vi "register status change event.vi"(11 "generate status number":i32=100) -> (3 "status number":i32)   [LabVIEW 2017, in "testcase-Basic-Function.lvclass"]
uses:
  testcase-Basic-Function.lvclass
  f9bca660-bddd-4266-99d8-d96952150cc2.vi
  src/user.lib/_NEVSTOP/Communicable State Machine(CSM)/Communicable State Machine.lvlib
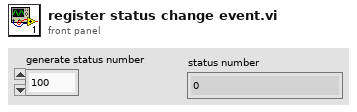
[diagram p1: front panel]
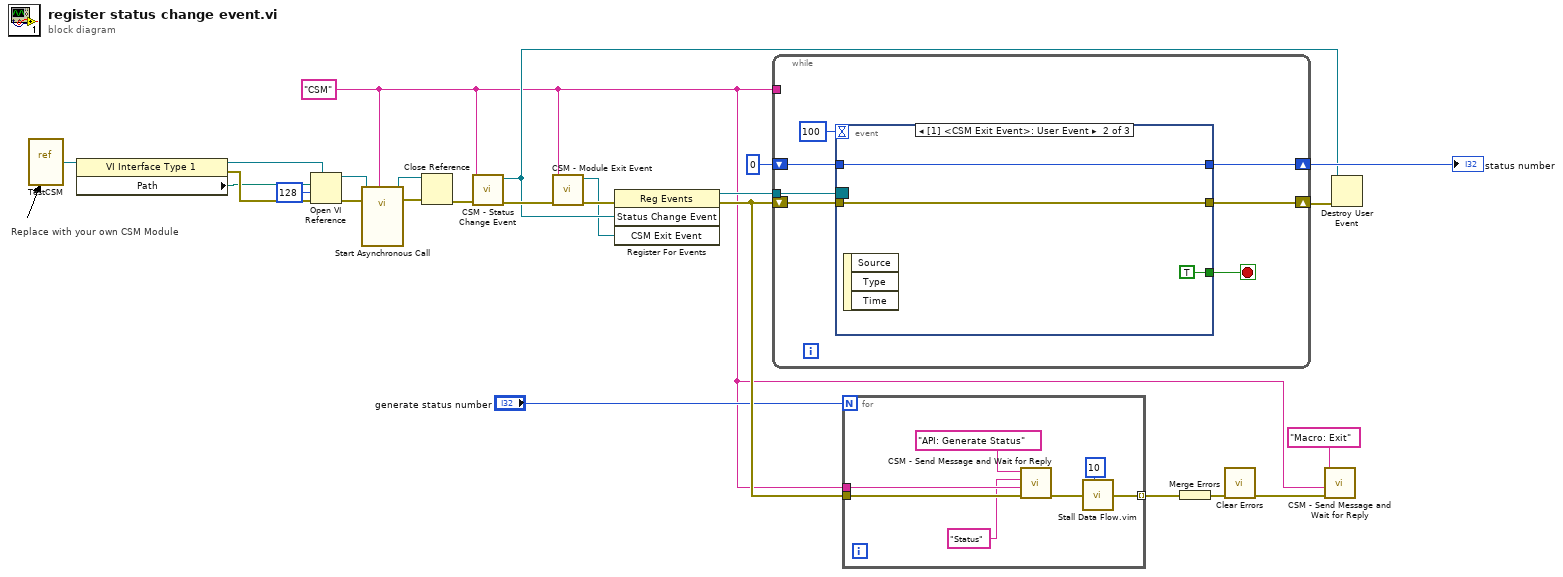
[diagram p0: block diagram]
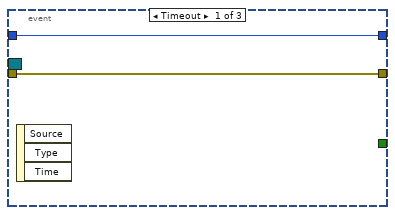
[diagram p2: hidden frame]
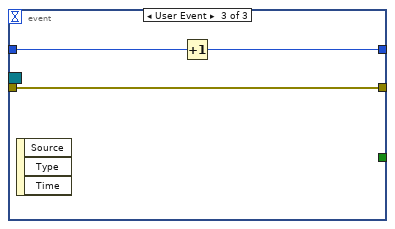
[diagram p3: hidden frame]
diagram:
  w3 = "CSM" ("Name(\"\" to use uuid)")
  # "Replace with your own CSM Module"
  n1 = vi-ref "TestCSM.vi"() -> (w18:refnum<vi>)
  n2 = property class="VI Interface Type 1"(reference=w18) -> (reference out=w22:refnum<vi>, error out=w20:errorcluster, "Path"=w19:path)  [unwired: 1 in]
  n3 = Open VI Reference(type specifier VI Refnum (for type only)=w22, vi path=w19, options=128, error in (no error)=w20) -> (vi reference=w21:refnum<vi>, error out=w17:errorcluster)  [unwired: 2 in]
  n4 = call-by-ref "Start Asynchronous Call"(reference=w21, error in=w17, "Name(\"\" to use uuid)"=w3) -> (reference out=w24:refnum<vi>, error out=w23:errorcluster)  [unwired: 11 in]
  n5 = Close Reference(reference=w24, error in (no error)=w23) -> (error out=w16:errorcluster)
  n6 = call "CSM - Status Change Event.vi"("Error in"=w16, "CSM Module"=w3) -> ("Error out"=w15:errorcluster, "Status Change Event"=w5:refnum<user-event>)  [unwired: 8 in]
  n7 = call "CSM - Module Exit Event.vi"("Error in"=w15, "Name(\"\" to use uuid) in"=w3) -> ("Error out"=w4:errorcluster, "CSM Exit Event"=w2:refnum<user-event>)  [unwired: 8 in]
  n8 = register-events(error in=w4, w5, w2) -> (reference out=w14:refnum<event-registration>, error out=w13:errorcluster)  [unwired: 1 in]
  n9 = while {
    tunnel: w14 -> [w32]
    tunnel: w3 -> [_]
    shift-right: [w28] -> w7
    shift-left: 0 -> [w30]
    shift-right: [w27] -> w6
    shift-left: w13 -> [w31]
    stop <- w26 stop-if-true
    n10 = event shown="[1] <CSM Exit Event>: User Event" {
      selector: w32 -> [_ _ _]
      dyn-events: _ -> [_ _ _]
      timeout: 100 -> [_ _ _]
      tunnel: w31 -> [w33 w36 w38]
      tunnel: w30 -> [w34 w37 w40]
      tunnel: [w34 w37 w39] -> w28
      tunnel: [w33 w36 w38] -> w27
      tunnel: [_ TRUE _] -> w26
      event Timeout {
        n11 = event-data() -> ()  [unwired: 1 in, 3 out]
      }
      event User Event {
        n12 = event-data() -> ()  [unwired: 1 in, 3 out]
      }
      event User Event {
        n13 = event-data() -> ()  [unwired: 1 in, 3 out]
        n14 = Increment(x=w40) -> (x+1=w39:i32)
      }
    }
  }
  "status number" <- w7
  n15 = for {
    N: "generate status number" -> [_]
    tunnel: w13 -> [w47]
    tunnel: w3 -> [w46]
    tunnel: [w42] -> w11 mode=indexing
    n16 = call "CSM - Send Message and Wait for Reply.vi"("Error In (no error)"=w47, "Target Module"=w46, "Arguments (\"\")"="Status" ("Arguments (\"\")"), "State"="API: Generate Status") -> ("error out"=w43:errorcluster)  [unwired: 5 in, 2 out]
    n17 = call "Stall Data Flow.vim"("value in"=w43, "milliseconds to wait"=10) -> ("value out"=w42:errorcluster)  [unwired: 1 out]
  }
  n18 = Merge Errors(w11) -> (w10:errorcluster)
  n19 = call <vilib>:"Clear Errors.vi"("error in (no error)"=w10) -> ("error out"=w1:errorcluster)  [unwired: 5 in, 1 out]
  n20 = call "CSM - Send Message and Wait for Reply.vi"("Error In (no error)"=w1, "Target Module"=w3, "State"="Macro: Exit") -> ()  [unwired: 6 in, 3 out]
  n21 = Destroy User Event(user event=w5, error in=w6) -> ()  [unwired: 1 out]
